vi "test Alternating Cell Background Color.vi"(11 "Test Case In":refnum<class "Test Cases.lvclass">) -> (0 "error out":errorcluster, 3 "Test Case Out":refnum<class "Test Cases.lvclass">)   [LabVIEW 2024, in "Test Cases.lvclass"]
uses:
  Test Cases.lvclass
  Test Cases.lvclass/Test Cases.ctl
  source/Grid/SourceGrid.lvclass
  <vilib>/Astemes/LUnit/Test Case.lvclass
  source/Cells/Cell/Cell.lvclass
  source/System.Drawing.Color.ctl
  source/SourceGrid.lvlib
  source/Views/Cell View Alternating Back Color/Cell View Alternating Back Color.lvclass
  C:/Program Files/National Instruments/LabVIEW 2025/vi.lib/Astemes/LUnit/Test Case.lvclass
  C:/Program Files/National Instruments/LabVIEW 2025/vi.lib/Astemes/LUnit/LUnit Runnable.lvclass
  D:/git/Sourcegrid-LabVIEW/tests/Tests/Test Cases.lvclass
  D:/git/Sourcegrid-LabVIEW/source/Views/Cell View/Cell View.lvclass
  D:/git/Sourcegrid-LabVIEW/source/Views/Cell View Alternating Back Color/Cell View Alternating Back Color.lvclass
  D:/git/Sourcegrid-LabVIEW/dll/SourceGrid.dll
  dll/SourceGrid.dll
panel:
  in  "Grid Container":refnum<k24>(container)
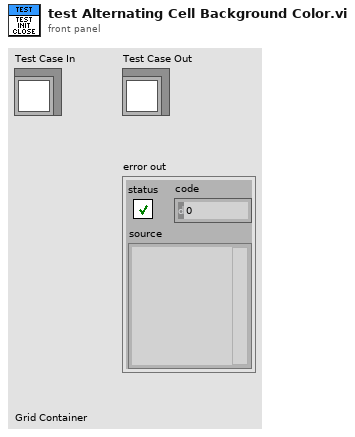
[diagram p1: front panel]
types:
  T1 = typedef "SourceGrid.lvlib/System.Drawing.Color.ctl" = enum16{"AliceBlue", "AntiqueWhite", "Aqua", "Aquamarine", "Azure", "Beige", "Bisque", "Black", "BlanchedAlmond", "Blue", "BlueViolet", "Brown", "BurlyWood", "CadetBlue", "Chartreuse", "Chocolate", "Coral", "CornflowerBlue", "Cornsilk", "Crimson", "Cyan", "DarkBlue", "DarkCyan", "DarkGoldenrod", "DarkGray", "DarkGreen", "DarkKhaki", "DarkMagenta", "DarkOliveGreen", "DarkOrange", "DarkOrchid", "DarkRed", "DarkSalmon", "DarkSeaGreen", "DarkSlateBlue", "DarkSlateGray", "DarkTurquoise", "DarkViolet", "DeepPink", "DeepSkyBlue", "DimGray", "DodgerBlue", "Firebrick", "FloralWhite", "ForestGreen", "Fuchsia", "Gainsboro", "GhostWhite", "Gold", "Goldenrod", "Gray", "Green", "GreenYellow", "Honeydew", "HotPink", "IndianRed", "Indigo", "Ivory", "Khaki", "Lavender", "LavenderBlush", "LawnGreen", "LemonChiffon", "LightBlue", "LightCoral", "LightCyan", "LightGoldenrodYellow", "LightGray", "LightGreen", "LightPink", "LightSalmon", "LightSeaGreen", "LightSkyBlue", "LightSlateGray", "LightSteelBlue", "LightYellow", "Lime", "LimeGreen", "Linen", "Magenta", "Maroon", "MediumAquamarine", "MediumBlue", "MediumOrchid", "MediumPurple", "MediumSeaGreen", "MediumSlateBlue", "MediumSpringGreen", "MediumTurquoise", "MediumVioletRed", "MidnightBlue", "MintCream", "MistyRose", "Moccasin", "NavajoWhite", "Navy", "OldLace", "Olive", "OliveDrab", "Orange", "OrangeRed", "Orchid", "PaleGoldenrod", "PaleGreen", "PaleTurquoise", "PaleVioletRed", "PapayaWhip", "PeachPuff", "Peru", "Pink", "Plum", "PowderBlue", "Purple", "Red", "RosyBrown", "RoyalBlue", "SaddleBrown", "Salmon", "SandyBrown", "SeaGreen", "SeaShell", "Sienna", "Silver", "SkyBlue", "SlateBlue", "SlateGray", "Snow", "SpringGreen", "SteelBlue", "Tan", "Teal", "Thistle", "Tomato", "Transparent", "Turquoise", "Violet", "Wheat", "White", "WhiteSmoke", "Yellow"}
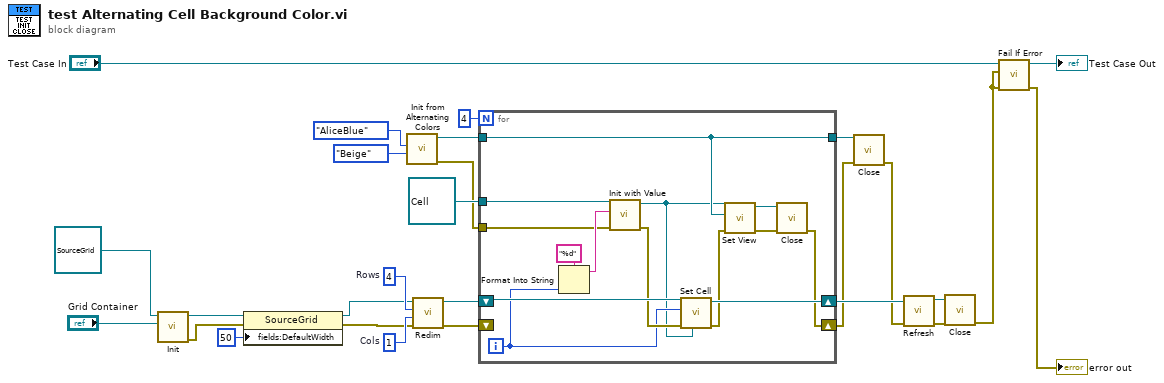
[diagram p0: block diagram]
diagram:
  w23 = 1  # Cols
  w24 = 4  # Rows
  n1 = call-dynamic "Init.vi"("Sourcegrid Container"="Grid Container", "Grid in"=refnum<class "SourceGrid.lvclass"> refnum) -> ("error out"=w9:errorcluster, "Grid out"=w20:refnum<class "SourceGrid.lvclass">)  [unwired: 8 in]
  n2 = property class="SourceGrid"(reference=w20, error in=w9, "fields:DefaultWidth"=50 ("DefaultWidth")) -> (reference out=w19:refnum<class "SourceGrid.lvclass">, error out=w18:errorcluster)
  n3 = call "Init from Alternating Colors.vi"("Color Not Equal"=System.Drawing.Color."Beige", "Color Equal"=System.Drawing.Color."AliceBlue") -> ("error out"=w5:errorcluster, "Cell View Alternating Back Color out"=w4:refnum<class "Cell View Alternating Back Color.lvclass">)  [unwired: 8 in]
  n4 = call "Redim.vi"("error in"=w18, "Columns"=w23, "Rows"=w24, "Sourcegrid in"=w19) -> ("error out"=w16:errorcluster, "Sourcegrid out"=w14:refnum<class "SourceGrid.lvclass">)  [unwired: 6 in]
  n5 = for {
    N: 4 -> [_]
    shift-right: [w38] -> w2
    shift-left: w16 -> [_]
    shift-right: [w41] -> w15
    shift-left: w14 -> [w40]
    tunnel: refnum<class "Cell.lvclass"> refnum ("Cell in") -> [w34]
    tunnel: w5 -> [w31]
    tunnel: w4 -> [w30]
    tunnel: [w30] -> w3
    i -> [w32]
    n6 = Format Into String(format string="%d", w32) -> (resulting string=w36:string)  [unwired: 2 in, 1 out]
    n7 = call-dynamic "Init with Value.vi"("error in"=w31, "Value"=w36, "Cell in"=w34) -> ("error out"=w35:errorcluster, "Cell out"=w28:refnum<class "Cell.lvclass">)  [unwired: 7 in]
    n8 = call "Set Cell.vi"("Cell"=w28, "error in"=w35, "Row"=w32, "Sourcegrid in"=w40) -> ("error out"=w33:errorcluster, "Sourcegrid out"=w41:refnum<class "SourceGrid.lvclass">)  [unwired: 6 in]
    n9 = call-dynamic "Set View.vi"("error in"=w33, "CellView"=w30, "Cell in"=w28) -> ("error out"=w29:errorcluster, "Cell out"=w39:refnum<class "Cell.lvclass">)  [unwired: 7 in]
    n10 = call-dynamic "Close.vi"("error in"=w29, "Cell in"=w39) -> ("error out"=w38:errorcluster)  [unwired: 8 in, 1 out]
  }
  n11 = call-dynamic "Close.vi"("error in"=w2, "Cell View Alternating Back Color in"=w3) -> ("error out"=w1:errorcluster)  [unwired: 8 in, 1 out]
  n12 = call "Refresh.vi"("error in"=w1, "SourceGrid in"=w15) -> ("error out"=w11:errorcluster, "SourceGrid out"=w12:refnum<class "SourceGrid.lvclass">)  [unwired: 8 in]
  n13 = call-dynamic "Close.vi"("error in"=w11, "Sourcegrid in"=w12) -> ("error out"=w22:errorcluster)  [unwired: 8 in, 1 out]
  n14 = call <vilib>:"Fail If Error.vi"("error in (no error)"=w22, "Assert error"=w22, "LUnit Test Case In"="Test Case In") -> ("error out"=→"error out":errorcluster, "LUnit Test Case Out"=→"Test Case Out":refnum<class "Test Cases.lvclass">)  [unwired: 7 in]
